vi "Test various functions.vi"() -> ()   [LabVIEW 2020]
uses:
  Controls/Sparameter cluster.ctl
  VNA-PNA.lvclass
  C:/Sandbox/RF Bench/Source Code/WiSpry Test Framework/Instruments/Instrument.lvclass
  Instrument.lvclass/Instrument.ctl
  Controls/S parm format enum.ctl
  Instrument.lvclass
  Vector Network Analyzer.lvclass
panel:
  in  "VISA resource name":refnum<visa-resource-name>="GPIB0::16::INSTR"
  out "Time elapsed":dbl
  out "S parameters":T1[](array[typedef])
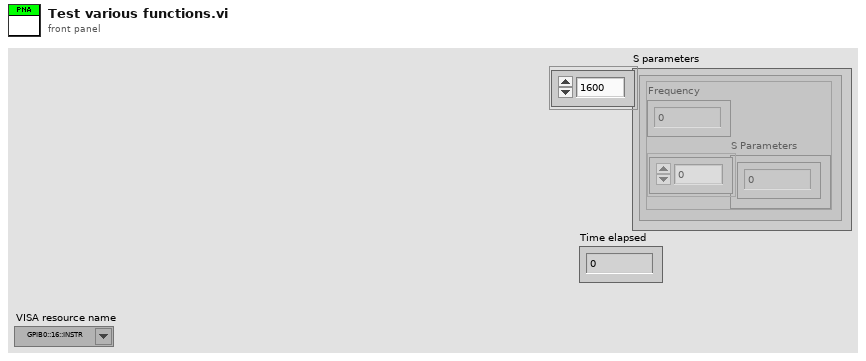
[diagram p1: front panel]
types:
  T1 = typedef "Vector Network Analyzer.lvclass/Sparameter cluster.ctl" = cluster{"Frequency":dbl, "S Parameters":cdb[]}
  T2 = enum16{"S11", "S21", "S31", "S41", "S22", "S12", "S32", "S42", "S33", "S13", "S23", "S43", "S44", "S14", "S24", "S34"}[]
  T3 = typedef "Vector Network Analyzer.lvclass/S parm format enum.ctl" = enum16{"Mag dB", "Mag", "Phase", "Smith", "Real", "Imag", "Group Delay", "SWR"}
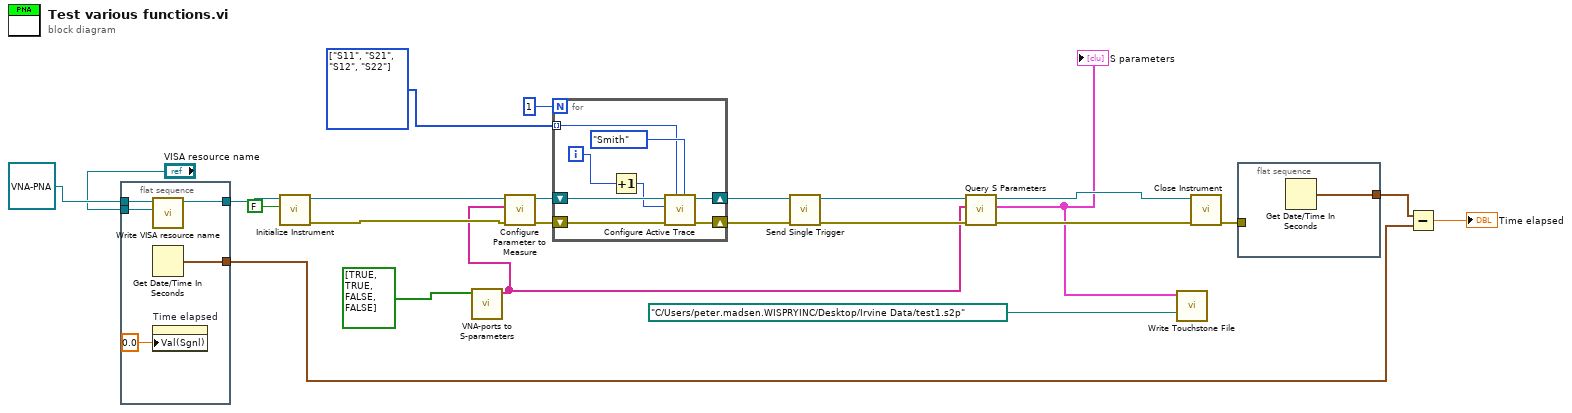
[diagram p0: block diagram]
diagram:
  w4 = T2 [enum."S11", enum."S21", enum."S12", enum."S22"] items=["S11", "S21", "S31", "S41", "S22", "S12", "S32", "S42", "S33", "S13", "S23", "S43", "S44", "S14", "S24", "S34"]
  n1 = flat-sequence {
    tunnel: refnum<class "VNA-PNA.lvclass"> refnum ("VNA-PNA.lvclass") -> [w29]
    tunnel: "VISA resource name" -> [w28]
    tunnel: [w27] -> w22
    tunnel: [w26] -> w19
    frame #0 {
      n2 = call "Write VISA resource name.vi"("VISA resource name"=w28, "Instrument in"=w29) -> ("Instrument out"=w27:refnum<class "VNA-PNA.lvclass">)  [unwired: 9 in]
      n3 = Get Date/Time In Seconds() -> (seconds since 1Jan1904=w26:timestamp)
      n4 = property on="Time elapsed" class="DigNum (strict)"("Val(Sgnl)"=0.0 ("Value (Signaling)")) -> ()  [unwired: 2 in, 2 out]
    }
  }
  n5 = call-dynamic "Initialize Instrument.vi"("Reset"=FALSE, "VNA-PNA in"=w22) -> ("error out"=w12:errorcluster, "VNA-PNA out"=w11:refnum<class "VNA-PNA.lvclass">)  [unwired: 8 in]
  n6 = call "VNA-ports to S-parameters.vi"("VNA ports"=bool[] [TRUE, TRUE, FALSE, FALSE]) -> ("Sparameters (string)"=w1:string[])  [unwired: 6 in, 4 out]
  n7 = call-dynamic "Configure Parameter to Measure.vi"("error in (no error)"=w12, "Sparameters (string)"=w1, "VNA-PNA in"=w11) -> ("error out"=w10:errorcluster, "VNA-PNA out"=w9:refnum<class "VNA-PNA.lvclass">)  [unwired: 7 in]
  n8 = for {
    N: 1 -> [_]
    shift-right: [w34] -> w7
    shift-left: w10 -> [w37]
    shift-right: [w35] -> w8
    shift-left: w9 -> [w36]
    tunnel: w4 -> [w32] mode=indexing
    i -> [w31]
    n9 = Increment(x=w31) -> (x+1=w30:i32)
    n10 = call-dynamic "Configure Active Trace.vi"("Format"=S_parm_format_enum."Smith", "S parameter"=w32, "error in (no error)"=w37, "Active Trace"=w30, "VNA-PNA in"=w36) -> ("error out"=w34:errorcluster, "VNA-PNA out"=w35:refnum<class "VNA-PNA.lvclass">)  [unwired: 5 in]
  }
  n11 = call-dynamic "Send Single Trigger.vi"("error in (no error)"=w7, "VNA-PNA in"=w8) -> ("error out"=w14:errorcluster, "VNA-PNA out"=w13:refnum<class "VNA-PNA.lvclass">)  [unwired: 8 in]
  n12 = call-dynamic "Query S Parameters.vi"("error in (no error)"=w14, "Sparameters (string)"=w1, "VNA-PNA in"=w13) -> ("error out"=w15:errorcluster, "S parameters"=w6:T1[], "VNA-PNA out"=w16:refnum<class "VNA-PNA.lvclass">)  [unwired: 6 in]
  "S parameters" <- w6
  n13 = call "Write Touchstone File.vi"("File Path"=path "C:/Users/peter.madsen.WISPRYINC/Desktop/Irvine Data/test1.s2p", "Sparameters"=w6) -> ()  [unwired: 9 in, 1 out]
  n14 = call-dynamic "Close Instrument.vi"("error in (no error)"=w15, "VNA-PNA in"=w16) -> ("error out"=w17:errorcluster)  [unwired: 8 in, 1 out]
  n15 = flat-sequence {
    tunnel: [w38] -> w20
    tunnel: w17 -> [_]
    frame #0 {
      n16 = Get Date/Time In Seconds() -> (seconds since 1Jan1904=w38:timestamp)
    }
  }
  n17 = Subtract(x=w20, y=w19) -> (x-y=→"Time elapsed":dbl)
